vi "SIPO.vi"(5 "Frequency":dbl, 6 "Serial":bool) -> (0 "Q4":bool, 1 "Q3":bool, 2 "Q2":bool, 3 "Q1":bool)   [LabVIEW 2018]
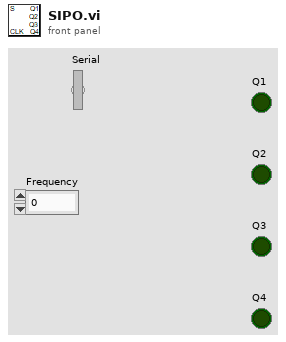
[diagram p1: front panel]
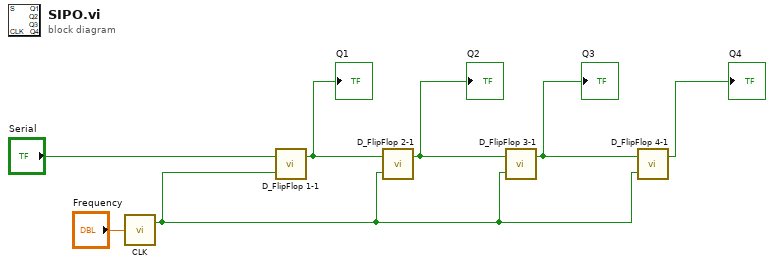
[diagram p0: block diagram]
diagram:
  n1 = call "CLK.vi"("Frequency"="Frequency") -> ("CLK"=w1:bool)  [unwired: 1 out]
  n2 = call "D_FlipFlop 1-1.vi"("CLK"=w1, "D"="Serial") -> ("Q"=w6:bool)  [unwired: 1 out]
  "Q1" <- w6
  n3 = call "D_FlipFlop 2-1.vi"("CLK"=w1, "D"=w6) -> ("Q"=w5:bool)  [unwired: 1 out]
  "Q2" <- w5
  n4 = call "D_FlipFlop 3-1.vi"("CLK"=w1, "D"=w5) -> ("Q"=w3:bool)  [unwired: 1 out]
  "Q3" <- w3
  n5 = call "D_FlipFlop 4-1.vi"("CLK"=w1, "D"=w3) -> ("Q"=→"Q4":bool)  [unwired: 1 out]
